vi "Send Single Trigger.vi"(8 "error in (no error)":errorcluster, 11 "VNA-FieldFox in":refnum<class "VNA-FieldFox.lvclass">) -> (0 "error out":errorcluster, 3 "VNA-FieldFox out":refnum<class "VNA-FieldFox.lvclass">)   [LabVIEW 2020, in "VNA-FieldFox.lvclass"]
doc: "Sent a single trigger for the VNA. It uses the OPC command to wait until completion.\nIt will use (sweeptime * N average * N ports) for the VISA timeout."
uses:
  VNA-FieldFox.lvclass
  C:/Sandbox/Git_Sandbox/WiSpry Test Framework source code (LV20)/WiSpry Test Framework/Instruments/Instrument.lvclass
  Instrument.lvclass/Instrument.ctl
  <instrlib>/Agilent N99XX Series/Public/Data/Low Level/Initiate (Continuous).vi
  <instrlib>/Agilent N99XX Series/Public/Data/Low Level/Initiate (Immediate).vi
  <instrlib>/Agilent N99XX Series/Agilent N99XX Series.lvlib
  Instrument.lvclass
panel:
  out "Numeric":i32
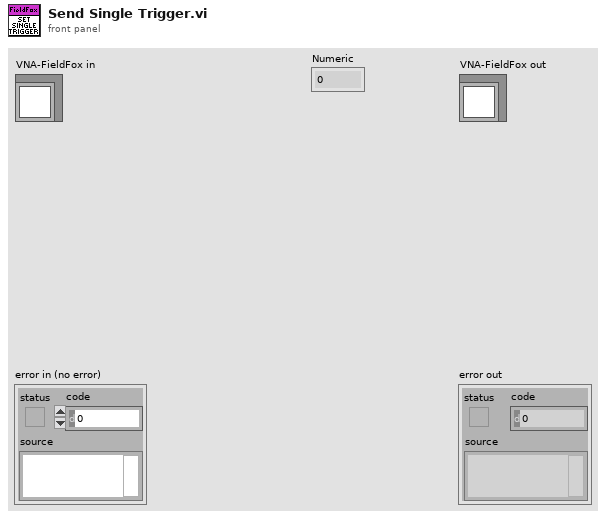
[diagram p1: front panel]
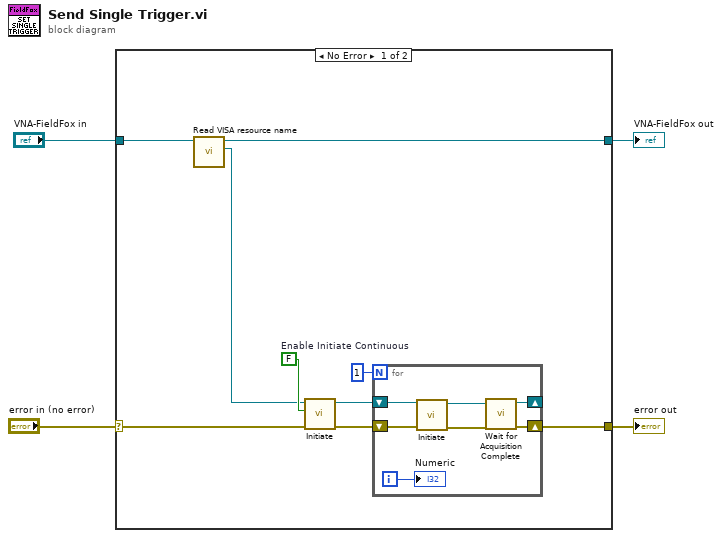
[diagram p0: block diagram]
diagram:
  n1 = case shown="No Error" "error in (no error)" {
    selector: "error in (no error)" -> [w9 w22]
    tunnel: [w8 w22] -> w3
    tunnel: [w6 w21] -> w2
    tunnel: "VNA-FieldFox in" -> [w7 w21]
    frame No Error {
      w13 = FALSE  # Enable Initiate Continuous
      n2 = call "Read VISA resource name.vi"("Instrument in"=w7) -> ("VISA resource name"=w5:refnum<visa-resource-name>, "Instrument out"=w6:refnum<class "VNA-FieldFox.lvclass">)  [unwired: 9 in]
      n3 = call-poly <instrlib>:"Initiate.vi"("error in (no error)"=w9, "Enable Initiate Continuous (T: Enable)"=w13, "VISA resource name"=w5) -> ("error out"=w10:errorcluster, "VISA resource name out"=w11:refnum<visa-resource-name>)  [unwired: 7 out]
      n4 = for {
        N: 1 -> [_]
        shift-right: [w15] -> w8
        shift-left: w10 -> [w17]
        shift-right: [w16] -> _
        shift-left: w11 -> [w18]
        i -> [w14]
        n5 = call-poly <instrlib>:"Initiate.vi"("error in (no error)"=w17, "VISA resource name"=w18) -> ("error out"=w19:errorcluster, "VISA resource name out"=w20:refnum<visa-resource-name>)  [unwired: 8 out]
        n6 = call <instrlib>:"Wait for Acquisition Complete.vi"("error in (no error)"=w19, "VISA resource name"=w20) -> ("error out"=w15:errorcluster, "VISA resource name out"=w16:refnum<visa-resource-name>)  [unwired: 1 in, 7 out]
        "Numeric" <- w14
      }
    }
    frame Error {
    }
  }
  "error out" <- w3
  "VNA-FieldFox out" <- w2
